vi "Start or restart timer.vi"(8 "error in (no error)":errorcluster, 11 "Timer name":string) -> (0 "error out":errorcluster)   [LabVIEW 2021, in "Named Timers.lvlib"]
uses:
  Named Timers.lvlib
  Timer Cluster.ctl
  Timer global variable.vi
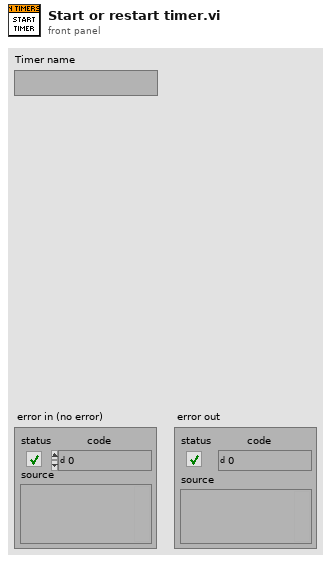
[diagram p1: front panel]
types:
  T1 = typedef "Named Timers.lvlib/Timer Cluster.ctl" = cluster{"Name":string, "Start time (ms)":u32}
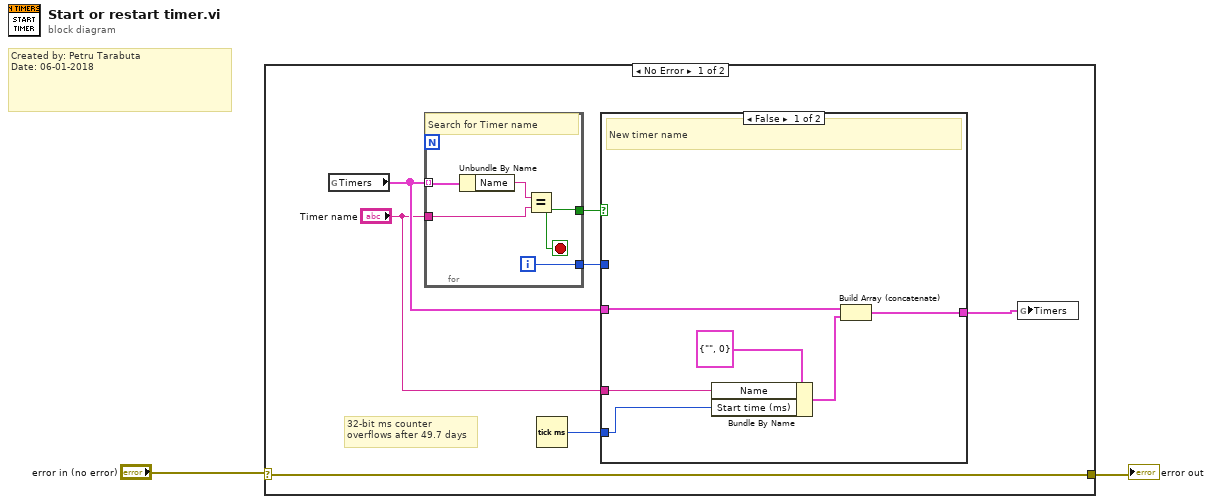
[diagram p0: block diagram]
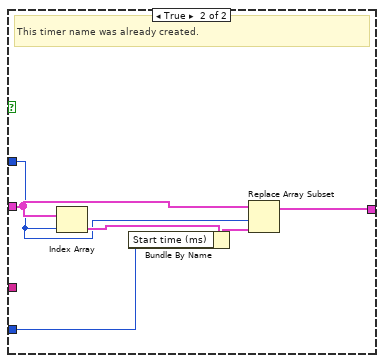
[diagram p2: hidden frame]
diagram:
  # "Created by: Petru Tarabuta\nDate: 06-01-2018"
  n1 = case shown="No Error" "error in (no error)" {
    selector: "error in (no error)" -> [w9 w27]
    tunnel: [w9 w27] -> w1
    frame No Error {
      # "32-bit ms counter\noverflows after 49.7 days"
      n2 = global read "Timer global variable.vi" "Timers"() -> (w7:T1[])
      n3 = for {
        tunnel: w7 -> [w26] mode=indexing
        tunnel: "Timer name" -> [w24]
        tunnel: [w23] -> w8
        tunnel: [w22] -> w4
        i -> [w22]
        stop <- w23 stop-if-true
        # "Search for Timer name"
        n4 = Unbundle By Name(w26) -> ("Name"=w25:string)
        n5 = Equal?(x=w25, y=w24) -> (x = y?=w23:bool)
      }
      n6 = Tick Count (ms)() -> (millisecond timer value=w3:u32)
      n7 = case shown="False" w8 {
        tunnel: w7 -> [w15 w19]
        tunnel: "Timer name" -> [w13 _]
        tunnel: [w11 w16] -> w5
        tunnel: w4 -> [_ w18]
        tunnel: w3 -> [w10 w20]
        frame False {
          # "New timer name"
          n8 = Bundle By Name(cluster=T1 {"Name"="", "Start time (ms)"=0} ("Timer Cluster"), "Name"=w13, "Start time (ms)"=w10) -> (w12:T1)
          n9 = Build Array (concatenate)(w15, w12) -> (w11:T1[])
        }
        frame True {
          # "This timer name was already created."
          n10 = Index Array(array=w19, index=w18) -> (element=w21:T1)
          n11 = Bundle By Name(cluster=w21, "Start time (ms)"=w20) -> (w17:T1)
          n12 = Replace Array Subset(array=w19, new element=w17, index=w18) -> (w16:T1[])
        }
      }
      n13 = global write "Timer global variable.vi" "Timers"(w5) -> ()
    }
    frame Error {
    }
  }
  "error out" <- w1
